vi "Correct_Alone_Problem_Point-1.vi"(1 "[IN] # of Prob\nlem Point Inside":i32, 2 "[IN] # of Longest track\nInside the Group of Tracks":i32, 3 "error IN":errorcluster, 4 "[IN] Still connected\ntracks in group":T2) -> (5 "[OUT] Clusters for Re\nconstructed Tracks":T1, 8 "error OUT":errorcluster)   [LabVIEW 2013]
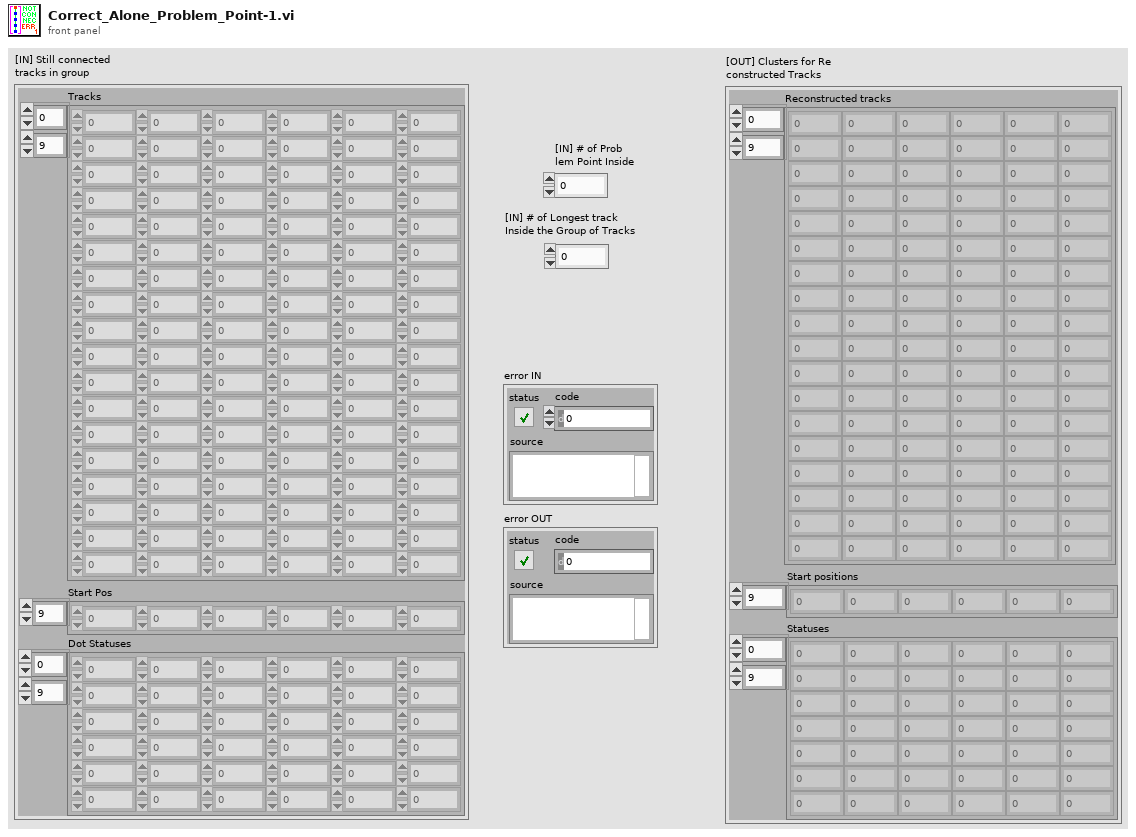
[diagram p1: front panel]
types:
  T1 = cluster{"Reconstructed tracks":dbl[][], "Start positions":i32[], "Statuses":i16[][]}
  T2 = cluster{"Tracks":dbl[][], "Start Pos":i32[], "Dot Statuses":i16[][]}
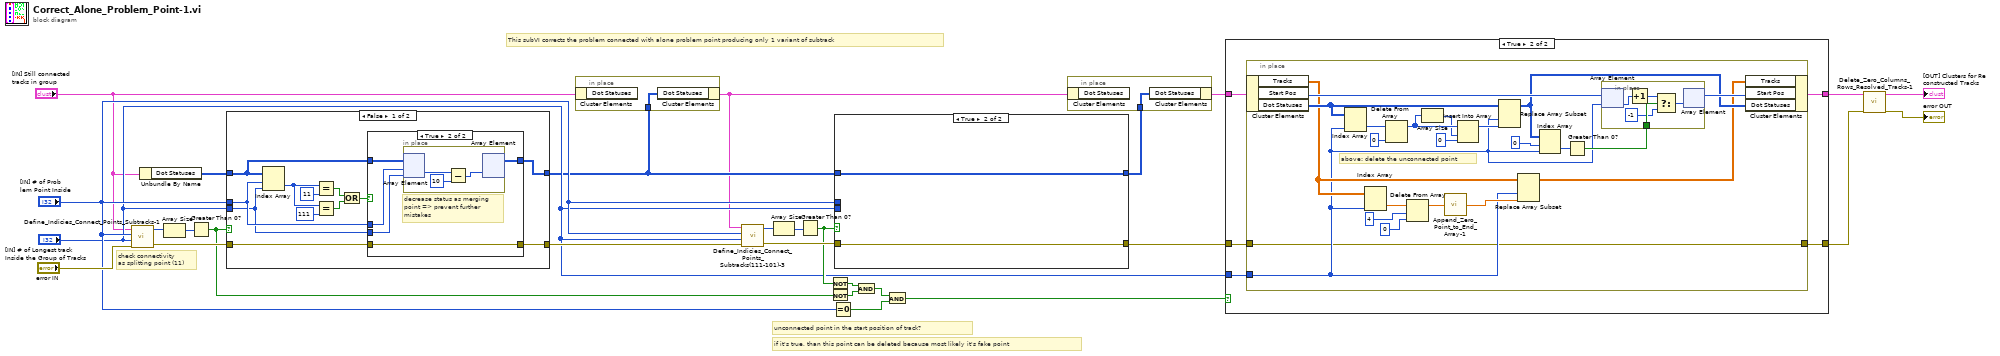
[diagram p0: block diagram]
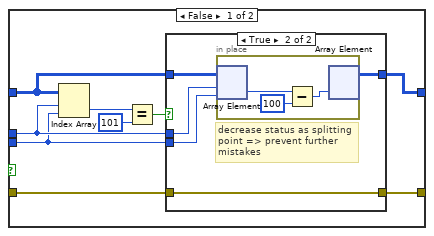
[diagram p3: hidden frame]
diagram:
  # "if it's true, than this point can be deleted because most likely it's fake point"
  # "unconnected point in the start position of track?"
  # "check connectivity \nas splitting point (11)"
  # "This subVI corrects the problem connected with alone problem point producing only 1 variant of subtrack"
  n1 = call "Define_Indicies_Connect_Points_Subtracks-1.vi"("error IN"="error IN", "[IN] Index of track with\n(problem displacement)"="[IN] # of Longest track\nInside the Group of Tracks", "[IN] Index of problem\ndisplacement inside track"="[IN] # of Prob\nlem Point Inside", "[IN] Track group"="[IN] Still connected\ntracks in group") -> ("error OUT"=w24:errorcluster, "[OUT] Index of connected\ntracks with problem dot"=w27:i32[])  [unwired: 1 out]
  n2 = Unbundle By Name("[IN] Still connected\ntracks in group") -> ("Dot Statuses"=w25:i16[][])
  n3 = Array Size(array=w27) -> (size(s)=w26:i32)
  n4 = Greater Than 0?(x=w26) -> (x > 0?=w18:bool)
  n5 = case shown="False" w18 {
    tunnel: w25 -> [w34 w52]
    tunnel: w24 -> [w30 w51]
    tunnel: [w31 w52] -> w2
    tunnel: "[IN] # of Prob\nlem Point Inside" -> [w33 _]
    tunnel: "[IN] # of Longest track\nInside the Group of Tracks" -> [w32 _]
    tunnel: [w29 w51] -> w23
    frame False {
      n6 = Index Array(array=w34, index (row)=w33, index (col)=w32) -> (element=w38:i16)
      n7 = Equal?(x=w38, y=i16 11) -> (x = y?=w37:bool)
      n8 = Equal?(x=w38, y=i16 111) -> (x = y?=w36:bool)
      n9 = Or(x=w37, y=w36) -> (x .or. y?=w35:bool)
      n10 = case shown="True" w35 {
        tunnel: w34 -> [w42 w47]
        tunnel: w33 -> [_ w46]
        tunnel: w32 -> [_ w45]
        tunnel: [w42 w44] -> w31
        tunnel: w30 -> [w41 w43]
        tunnel: [w41 w43] -> w29
        frame False {
          # "only merging event can occur"
        }
        frame True {
          # "decrease status as merging\npoint => prevent further \nmistakes"
          n11 = in-place {
            n12 = in-place-array #1(w47, w46, w45) -> (w50:i16)
            n13 = Subtract(x=w50, y=i16 10) -> (x-y=w48:i16)
            n14 = in-place-array #1(w48) -> (w44:i16[][])  [unwired: 2 out]
          }
        }
      }
    }
    frame True {
    }
  }
  n15 = in-place {
    in-place-border: w2 -> [w53]
    n16 = in-place-cluster #2("[IN] Still connected\ntracks in group") -> ()  [unwired: 1 out]
    n17 = in-place-cluster #2("Dot Statuses"=w53) -> (w1:T2)
  }
  n18 = call "Define_Indicies_Connect_Points_Subtracks(111-101)-3.vi"("error IN"=w23, "[IN] Index of single track\n(problem displacement)"="[IN] # of Longest track\nInside the Group of Tracks", "[IN] Index of problem\ndisplacement inside track"="[IN] # of Prob\nlem Point Inside", "[IN] Track group"=w1) -> ("error OUT"=w20:errorcluster, "[OUT] Index of connected\ntracks with problem dot"=w21:i32[])  [unwired: 1 out]
  n19 = Array Size(array=w21) -> (size(s)=w22:i32)
  n20 = Greater Than 0?(x=w22) -> (x > 0?=w19:bool)
  n21 = Not(x=w19) -> (.not. x?=w17:bool)
  n22 = Not(x=w18) -> (.not. x?=w16:bool)
  n23 = Equal To 0?(x="[IN] # of Prob\nlem Point Inside") -> (x = 0?=w10:bool)
  n24 = case shown="True" w19 {
    tunnel: w2 -> [w60 w74]
    tunnel: w20 -> [w56 w73]
    tunnel: [w57 w74] -> w14
    tunnel: "[IN] # of Prob\nlem Point Inside" -> [w59 _]
    tunnel: "[IN] # of Longest track\nInside the Group of Tracks" -> [w58 _]
    tunnel: [w55 w73] -> w15
    frame False {
      n25 = Index Array(array=w60, index (row)=w59, index (col)=w58) -> (element=w61:i16)
      n26 = Equal?(x=w61, y=i16 101) -> (x = y?=w54:bool)
      n27 = case shown="True" w54 {
        tunnel: w60 -> [w64 w69]
        tunnel: w59 -> [_ w68]
        tunnel: w58 -> [_ w67]
        tunnel: [w64 w66] -> w57
        tunnel: w56 -> [w63 w65]
        tunnel: [w63 w65] -> w55
        frame False {
          # "or nothing"
          # "only splitting event can occur"
        }
        frame True {
          # "decrease status as splitting\npoint => prevent further \nmistakes"
          n28 = in-place {
            n29 = in-place-array #3(w69, w68, w67) -> (w72:i16)
            n30 = Subtract(x=w72, y=i16 100) -> (x-y=w70:i16)
            n31 = in-place-array #3(w70) -> (w66:i16[][])  [unwired: 2 out]
          }
        }
      }
    }
    frame True {
    }
  }
  n32 = And(x=w17, y=w16) -> (x .and. y?=w11:bool)
  n33 = And(x=w11, y=w10) -> (x .and. y?=w9:bool)
  n34 = in-place {
    in-place-border: w14 -> [w75]
    n35 = in-place-cluster #4(w1) -> ()  [unwired: 1 out]
    n36 = in-place-cluster #4("Dot Statuses"=w75) -> (w13:T2)
  }
  n37 = case shown="True" w9 {
    tunnel: w15 -> [w76 w81]
    tunnel: w13 -> [w77 w82]
    tunnel: "[IN] # of Longest track\nInside the Group of Tracks" -> [_ w80]
    tunnel: [w77 w79] -> w7
    tunnel: [w76 w78] -> w6
    frame False {
    }
    frame True {
      n38 = in-place {
        in-place-border: w81 -> [w83]
        in-place-border: w80 -> [w85]
        in-place-border: [w83] -> w78
        # "above: delete the unconnected point"
        n39 = in-place-cluster #5(w82) -> ("Tracks"=w87:dbl[][], "Start Pos"=w95:i32[], "Dot Statuses"=w102:i16[][])
        n40 = Index Array(array=w102, index (col)=w85) -> (element=w104:i16[])  [unwired: 1 in]
        n41 = Index Array(array=w87, index (col)=w85) -> (element=w91:dbl[])  [unwired: 1 in]
        n42 = Delete From Array(array=w104, index=0) -> (array with subset deleted=w100:i16[])  [unwired: 1 in, 1 out]
        n43 = Delete From Array(array=w91, length=4, index=0) -> (array with subset deleted=w90:dbl[])  [unwired: 1 out]
        n44 = Array Size(array=w100) -> (size(s)=w99:i32)
        n45 = call "Append_Zero_Point_to_End_Array-1.vi"("[IN] Array with \nDisplacements"=w90) -> ("[OUT] Array with \nAppended Point"=w86:dbl[])
        n46 = Insert Into Array(array=w100, index=w99, new element=i16 0 ("new element/subarray")) -> (w98:i16[])
        n47 = Replace Array Subset(array=w102, new element=w98, index (col)=w85) -> (w92:i16[][])  [unwired: 1 in]
        n48 = Replace Array Subset(array=w87, new element=w86, index (col)=w85) -> (w84:dbl[][])  [unwired: 1 in]
        n49 = Index Array(array=w92, index (row)=0 ("disabled index (row)"), index (col)=w85) -> (element=w96:i16)
        n50 = Greater Than 0?(x=w96) -> (x > 0?=w94:bool)
        n51 = in-place {
          in-place-border: w94 -> [w109]
          n52 = in-place-array #6(w95, w85) -> (w108:i32)
          n53 = Increment(x=w108) -> (x+1=w107:i32)
          n54 = Select(t=w107, s=w109, f=-1) -> (s? t:f=w106:i32)
          n55 = in-place-array #6(w106) -> (w93:i32[])  [unwired: 1 out]
        }
        n56 = in-place-cluster #5("Tracks"=w84, "Start Pos"=w93, "Dot Statuses"=w92) -> (w79:T2)
      }
    }
  }
  n57 = call "Delete_Zero_Columns_Rows_Resolved_Tracks-1.vi"("error IN"=w6, "[IN] Clusters for Re\nconstructed Tracks"=w7) -> ("error OUT"=→"error OUT":errorcluster, "[OUT] Clusters for Re\nconstructed Tracks"=→"[OUT] Clusters for Re\nconstructed Tracks":T1)  [unwired: 4 in]
